vi "ManualModeLidar.vi"(4 "LIDARControl":T1, 6 "error in":errorcluster, 7 "initialized \nsonar ray\narray":i32[](array[numeric]), 8 "MDF Image":T2, 9 "SubPosition":T3) -> (0 "error out":errorcluster, 1 "Collision\nWarning":bool, 2 "LIDAR Data (r:pixel b:degrees)":cluster{"Range":dbl, "Bearing":dbl}[](array[cluster]), 3 "LIDAR":picture)   [LabVIEW 2012]
doc: "This SubVI plots the simulated pixe lLIDAR data for the curretn MDF file given the robots current position"
uses:
  <vilib>/vision/Image Controls.llb/IMAQ Image.ctl
panel:
  # "This SubVI plots the pixelsonar data for the TunaSub's current position in the MDF file"
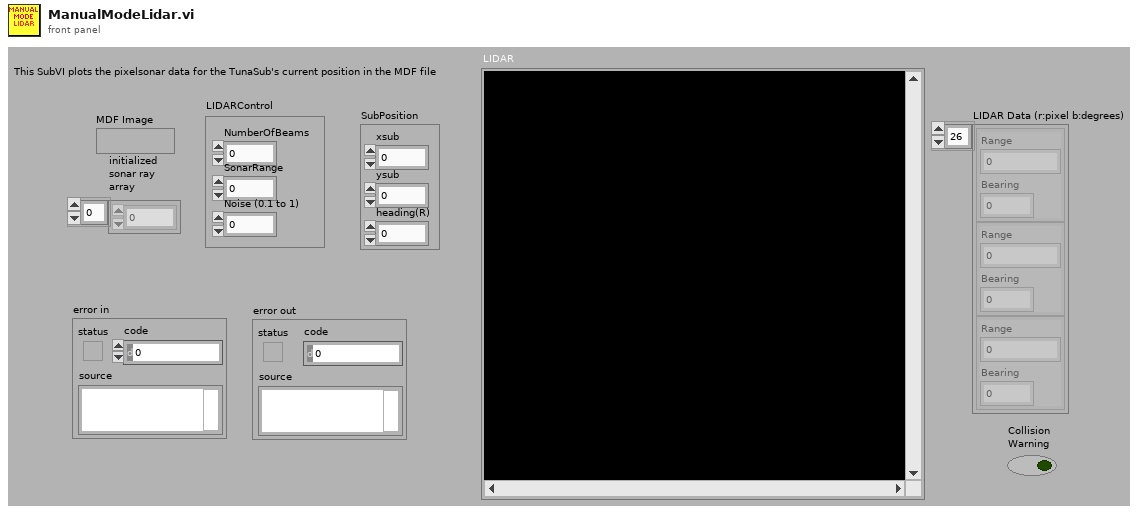
[diagram p1: front panel]
types:
  T1 = cluster{"NumberOfBeams":i32, "SonarRange":dbl, "Noise (0.1 to 1)":dbl}
  T2 = typedef "IMAQ Image.ctl" = refnum<image>
  T3 = cluster{"xsub":dbl, "ysub":dbl, "heading(R)":dbl}
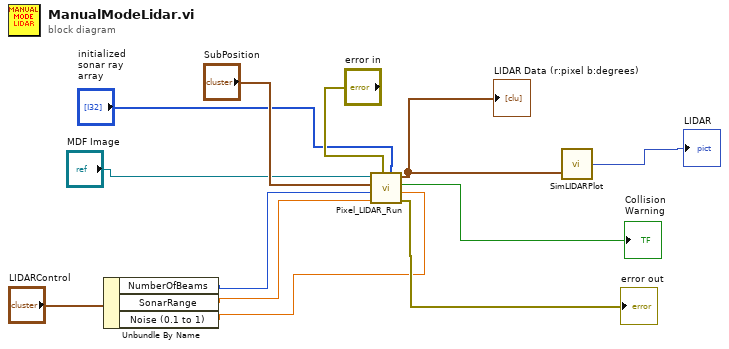
[diagram p0: block diagram]
diagram:
  n1 = Unbundle By Name("LIDARControl") -> ("NumberOfBeams"=w4:i32, "SonarRange"=w3:dbl, "Noise (0.1 to 1)"=w2:dbl)
  n2 = call "Pixel_LIDAR_Run.vi"("Noise (0.1 to 1)"=w2, "Initial\nSonarRay\nArray"="initialized \nsonar ray\narray", "error in (no error)"="error in", "SonarRange"=w3, "NumberOfBeams"=w4, "SubPosition"="SubPosition", "MDF Image In"="MDF Image") -> ("error out"=→"error out":errorcluster, "Collision\nWarning"=→"Collision\nWarning":bool, "Sonar Data (r:pixel b:degrees)"=w11:cluster{"Range":dbl, "Bearing":dbl}[])
  "LIDAR Data (r:pixel b:degrees)" <- w11
  n3 = call "SimLIDARPlot.vi"("data array [mag, phase (deg)]"=w11) -> ("SONAR"=→"LIDAR":picture)  [unwired: 1 in]
